vi "SmartSearch.vi"() -> ()   [LabVIEW 2015]
uses:
  <vilib>/NXT/Subs/MotorOutput.ctl
  <vilib>/NXT/Block Support/NXT_InputPort.ctl
  <vilib>/NXT/Dual Mode Library/Sensors/Light_On.vi
  <vilib>/NXT/Dual Mode Library/Motors/MotorReverse.vi
  <vilib>/NXT/Dual Mode Library/Waits/Wait_Num.vi
  <vilib>/NXT/Dual Mode Library/Motors/MotorOn.vi
  <vilib>/NXT/Dual Mode Library/Motors/MotorBrake.vi
  <vilib>/NXT/Dual Mode Library/Sensors/Sonar_cm.vi
panel:
  in  "정지":bool
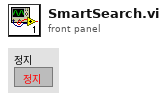
[diagram p1: front panel]
types:
  T1 = typedef "MotorOutput.ctl" = u8
  T2 = typedef "NXT_InputPort.ctl" = u32
  T3 = typedef "LVHSConnector.ctl" = refnum<class "BrickReference.lvclass">
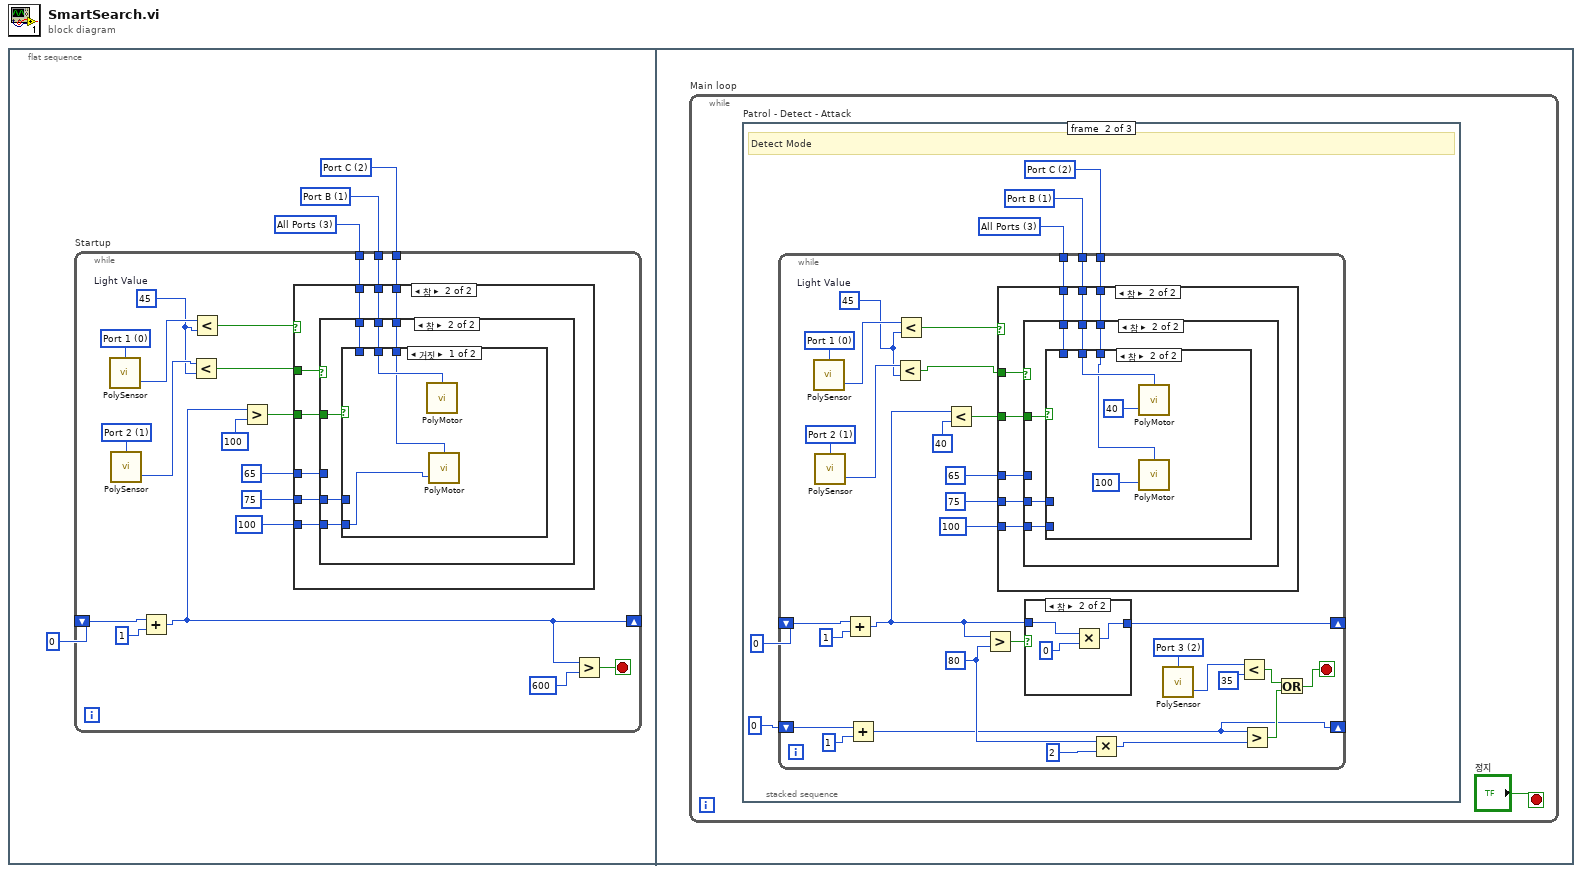
[diagram p0: block diagram]
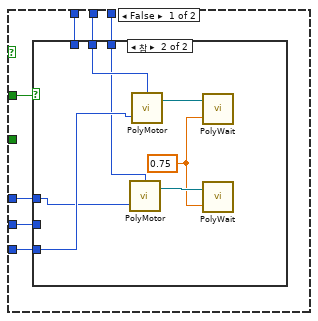
[diagram p2: hidden frame]
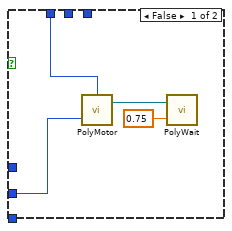
[diagram p3: hidden frame]
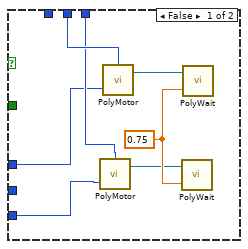
[diagram p4: hidden frame]
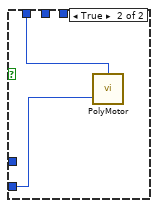
[diagram p5: hidden frame]
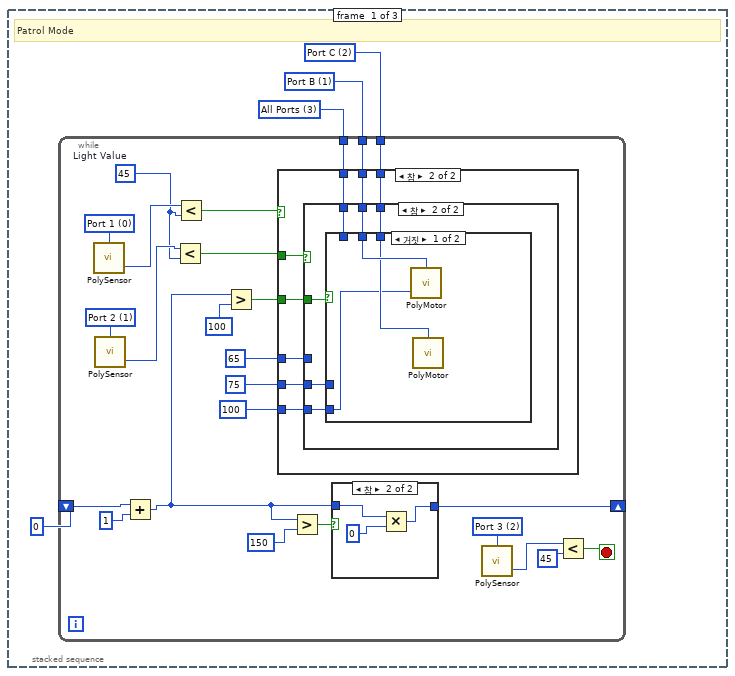
[diagram p6: hidden frame]
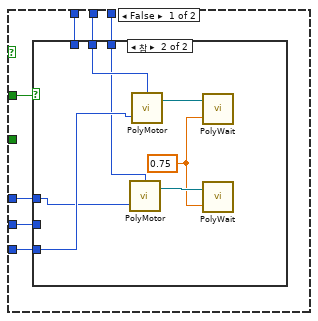
[diagram p8: hidden frame]
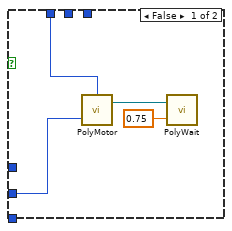
[diagram p9: hidden frame]
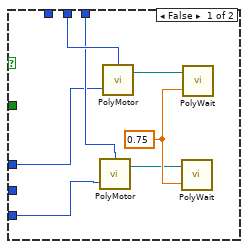
[diagram p10: hidden frame]
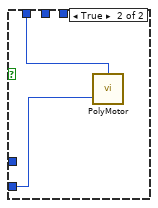
[diagram p11: hidden frame]
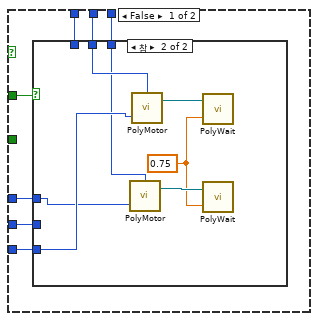
[diagram p13: hidden frame]
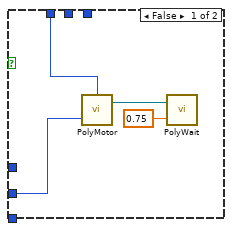
[diagram p14: hidden frame]
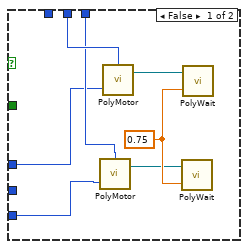
[diagram p15: hidden frame]
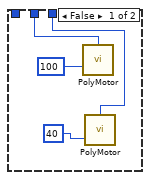
[diagram p16: hidden frame]
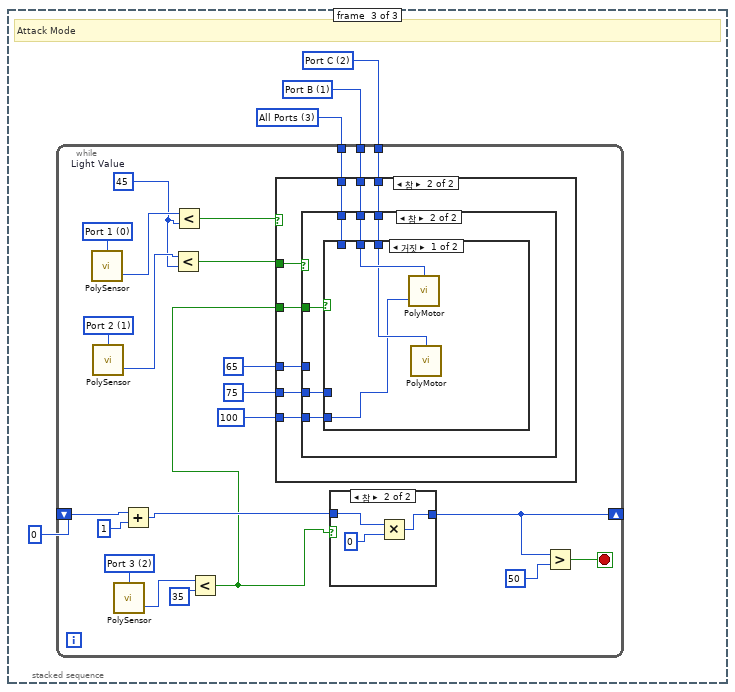
[diagram p17: hidden frame]
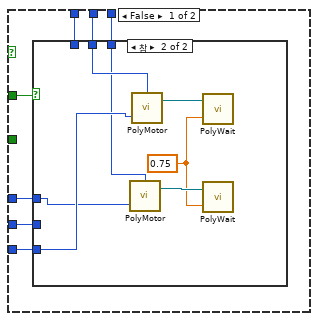
[diagram p19: hidden frame]
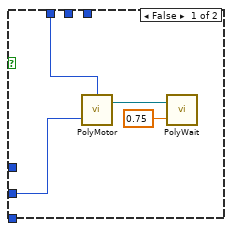
[diagram p20: hidden frame]
diagram:
  n1 = flat-sequence {
    frame #0 {
      w1 = T1 2 items=["Port A"=0, "Port B"=1, "Port C"=2, "Ports A & B"=4, "Ports A & C"=5, "Ports B & C"=6, "All Ports"=3] ("Output Port (All Ports)")
      w2 = T1 1 items=["Port A"=0, "Port B"=1, "Port C"=2, "Ports A & B"=4, "Ports A & C"=5, "Ports B & C"=6, "All Ports"=3] ("Output Port (All Ports)")
      w3 = T1 3 items=["Port A"=0, "Port B"=1, "Port C"=2, "Ports A & B"=4, "Ports A & C"=5, "Ports B & C"=6, "All Ports"=3] ("Output Port (All Ports)")
      n2 = while "Startup" {
        shift-right: [w7] -> _
        shift-left: i16 0 ("y") -> [w12]
        tunnel: w3 -> [w18]
        tunnel: w2 -> [w17]
        tunnel: w1 -> [w16]
        stop <- w6 stop-if-true
        w5 = i16 45  # Light Value
        w22 = T2 1 items=["Port 1", "Port 2", "Port 3", "Port 4"] ("Port (Port 3)")
        w24 = T2 0 items=["Port 1", "Port 2", "Port 3", "Port 4"] ("Port (Port 3)")
        n3 = call-poly <vilib>:"PolySensor.vi"("Port (Port 3)"=w24) -> ("Scaled Value"=w23:i16)  [unwired: 2 in, 1 out]
        n4 = call-poly <vilib>:"PolySensor.vi"("Port (Port 3)"=w22) -> ("Scaled Value"=w21:i16)  [unwired: 2 in, 1 out]
        n5 = Add(x=w12, y=i16 1) -> (x+y=w7:i16)
        n6 = Less?(x=w21, y=w5) -> (x < y?=w8:bool)
        n7 = Less?(x=w23, y=w5) -> (x < y?=w9:bool)
        n8 = Greater?(x=w7, y=i16 100) -> (0:w11:bool)
        n9 = case shown="참" w9 {
          tunnel: w8 -> [w31 w50]
          tunnel: w18 -> [w27 w49]
          tunnel: w17 -> [w26 w48]
          tunnel: w16 -> [w25 w47]
          tunnel: 75 ("Power (75)") -> [w30 w45]
          tunnel: 65 ("Power (75)") -> [w29 w43]
          tunnel: 100 ("Power (75)") -> [w28 w46]
          tunnel: w11 -> [_ w44]
          frame False {
            n10 = case shown="참" w31 {
              tunnel: w30 -> [w34 _]
              tunnel: w29 -> [_ w36]
              tunnel: w28 -> [_ w39]
              tunnel: w27 -> [w32 _]
              tunnel: w26 -> [_ w38]
              tunnel: w25 -> [_ w37]
              frame False {
                n11 = call-poly <vilib>:"PolyMotor.vi"("Power (75)"=w34, "Output Port (All Ports)"=w32) -> ("NXT/EV3"=w33:T3)  [unwired: 1 in, 1 out]
                n12 = call-poly <vilib>:"PolyWait.vi"("Time (1 sec)"=sgl 0.75, "NXT/EV3"=w33) -> ()  [unwired: 2 in, 1 out]
              }
              frame True {
                w40 = sgl 0.75 ("Time (1 sec)")
                n13 = call-poly <vilib>:"PolyMotor.vi"("Power (75)"=w36, "Output Port (All Ports)"=w37) -> ("NXT/EV3"=w41:T3)  [unwired: 1 in, 1 out]
                n14 = call-poly <vilib>:"PolyMotor.vi"("Power (75)"=w39, "Output Port (All Ports)"=w38) -> ("NXT/EV3"=w42:T3)  [unwired: 1 in, 1 out]
                n15 = call-poly <vilib>:"PolyWait.vi"("Time (1 sec)"=w40, "NXT/EV3"=w42) -> ()  [unwired: 2 in, 1 out]
                n16 = call-poly <vilib>:"PolyWait.vi"("Time (1 sec)"=w40, "NXT/EV3"=w41) -> ()  [unwired: 2 in, 1 out]
              }
            }
          }
          frame True {
            n17 = case shown="참" w50 {
              tunnel: w49 -> [_ w63]
              tunnel: w48 -> [w53 w62]
              tunnel: w47 -> [w52 w61]
              tunnel: w46 -> [w54 w59]
              tunnel: w45 -> [_ w60]
              tunnel: w44 -> [_ w58]
              tunnel: w43 -> [w51 _]
              frame False {
                w57 = sgl 0.75 ("Time (1 sec)")
                n18 = call-poly <vilib>:"PolyMotor.vi"("Power (75)"=w54, "Output Port (All Ports)"=w52) -> ("NXT/EV3"=w56:T3)  [unwired: 1 in, 1 out]
                n19 = call-poly <vilib>:"PolyMotor.vi"("Power (75)"=w51, "Output Port (All Ports)"=w53) -> ("NXT/EV3"=w55:T3)  [unwired: 1 in, 1 out]
                n20 = call-poly <vilib>:"PolyWait.vi"("Time (1 sec)"=w57, "NXT/EV3"=w56) -> ()  [unwired: 2 in, 1 out]
                n21 = call-poly <vilib>:"PolyWait.vi"("Time (1 sec)"=w57, "NXT/EV3"=w55) -> ()  [unwired: 2 in, 1 out]
              }
              frame True {
                n22 = case shown="거짓" w58 {
                  tunnel: w63 -> [_ w68]
                  tunnel: w62 -> [w66 _]
                  tunnel: w61 -> [w65 _]
                  tunnel: w60 -> [_ _]
                  tunnel: w59 -> [w64 w67]
                  frame False {
                    n23 = call-poly <vilib>:"PolyMotor.vi"("Port (All Ports)"=w66) -> ()  [unwired: 2 in, 2 out]
                    n24 = call-poly <vilib>:"PolyMotor.vi"("Power (75)"=w64, "Output Port (All Ports)"=w65) -> ()  [unwired: 1 in, 2 out]
                  }
                  frame True {
                    n25 = call-poly <vilib>:"PolyMotor.vi"("Power (75)"=w67, "Output Port (All Ports)"=w68) -> ()  [unwired: 1 in, 2 out]
                  }
                }
              }
            }
          }
        }
        n26 = Greater? ("보다 큼?")(x=w7, y=i16 600) -> (0:w6:bool)
      }
    }
    frame #1 {
      n27 = while "Main loop" {
        stop <- "정지" stop-if-true
        n28 = stacked-sequence "Patrol - Detect - Attack" {
          frame #0 {
            w70 = T1 2 items=["Port A"=0, "Port B"=1, "Port C"=2, "Ports A & B"=4, "Ports A & C"=5, "Ports B & C"=6, "All Ports"=3] ("Output Port (All Ports)")
            w71 = T1 1 items=["Port A"=0, "Port B"=1, "Port C"=2, "Ports A & B"=4, "Ports A & C"=5, "Ports B & C"=6, "All Ports"=3] ("Output Port (All Ports)")
            w72 = T1 3 items=["Port A"=0, "Port B"=1, "Port C"=2, "Ports A & B"=4, "Ports A & C"=5, "Ports B & C"=6, "All Ports"=3] ("Output Port (All Ports)")
            # "Patrol Mode"
            n29 = while {
              shift-right: [w79] -> _
              shift-left: i16 0 ("y") -> [w82]
              tunnel: w72 -> [w88]
              tunnel: w71 -> [w87]
              tunnel: w70 -> [w86]
              stop <- w81 stop-if-true
              w95 = T2 2 items=["Port 1", "Port 2", "Port 3", "Port 4"] ("Port (Port 3)")
              w96 = T2 1 items=["Port 1", "Port 2", "Port 3", "Port 4"] ("Port (Port 3)")
              w93 = i16 45  # Light Value
              w98 = T2 0 items=["Port 1", "Port 2", "Port 3", "Port 4"] ("Port (Port 3)")
              n30 = call-poly <vilib>:"PolySensor.vi"("Port (Port 3)"=w98) -> ("Scaled Value"=w97:i16)  [unwired: 2 in, 1 out]
              n31 = call-poly <vilib>:"PolySensor.vi"("Port (Port 3)"=w96) -> ("Scaled Value"=w94:i16)  [unwired: 2 in, 1 out]
              n32 = Add(x=w82, y=i16 1) -> (x+y=w77:i16)
              n33 = Less?(x=w94, y=w93) -> (x < y?=w74:bool)
              n34 = Less?(x=w97, y=w93) -> (x < y?=w75:bool)
              n35 = Greater?(x=w77, y=i16 100) -> (0:w80:bool)
              n36 = case shown="참" w75 {
                tunnel: w74 -> [w109 w128]
                tunnel: w88 -> [w105 w127]
                tunnel: w87 -> [w104 w126]
                tunnel: w86 -> [w103 w125]
                tunnel: 75 ("Power (75)") -> [w108 w123]
                tunnel: 65 ("Power (75)") -> [w107 w121]
                tunnel: 100 ("Power (75)") -> [w106 w124]
                tunnel: w80 -> [_ w122]
                frame False {
                  n37 = case shown="참" w109 {
                    tunnel: w108 -> [w112 _]
                    tunnel: w107 -> [_ w114]
                    tunnel: w106 -> [_ w117]
                    tunnel: w105 -> [w110 _]
                    tunnel: w104 -> [_ w116]
                    tunnel: w103 -> [_ w115]
                    frame False {
                      n38 = call-poly <vilib>:"PolyMotor.vi"("Power (75)"=w112, "Output Port (All Ports)"=w110) -> ("NXT/EV3"=w111:T3)  [unwired: 1 in, 1 out]
                      n39 = call-poly <vilib>:"PolyWait.vi"("Time (1 sec)"=sgl 0.75, "NXT/EV3"=w111) -> ()  [unwired: 2 in, 1 out]
                    }
                    frame True {
                      w118 = sgl 0.75 ("Time (1 sec)")
                      n40 = call-poly <vilib>:"PolyMotor.vi"("Power (75)"=w114, "Output Port (All Ports)"=w115) -> ("NXT/EV3"=w119:T3)  [unwired: 1 in, 1 out]
                      n41 = call-poly <vilib>:"PolyMotor.vi"("Power (75)"=w117, "Output Port (All Ports)"=w116) -> ("NXT/EV3"=w120:T3)  [unwired: 1 in, 1 out]
                      n42 = call-poly <vilib>:"PolyWait.vi"("Time (1 sec)"=w118, "NXT/EV3"=w120) -> ()  [unwired: 2 in, 1 out]
                      n43 = call-poly <vilib>:"PolyWait.vi"("Time (1 sec)"=w118, "NXT/EV3"=w119) -> ()  [unwired: 2 in, 1 out]
                    }
                  }
                }
                frame True {
                  n44 = case shown="참" w128 {
                    tunnel: w127 -> [_ w141]
                    tunnel: w126 -> [w131 w140]
                    tunnel: w125 -> [w130 w139]
                    tunnel: w124 -> [w132 w137]
                    tunnel: w123 -> [_ w138]
                    tunnel: w122 -> [_ w136]
                    tunnel: w121 -> [w129 _]
                    frame False {
                      w135 = sgl 0.75 ("Time (1 sec)")
                      n45 = call-poly <vilib>:"PolyMotor.vi"("Power (75)"=w132, "Output Port (All Ports)"=w130) -> ("NXT/EV3"=w134:T3)  [unwired: 1 in, 1 out]
                      n46 = call-poly <vilib>:"PolyMotor.vi"("Power (75)"=w129, "Output Port (All Ports)"=w131) -> ("NXT/EV3"=w133:T3)  [unwired: 1 in, 1 out]
                      n47 = call-poly <vilib>:"PolyWait.vi"("Time (1 sec)"=w135, "NXT/EV3"=w134) -> ()  [unwired: 2 in, 1 out]
                      n48 = call-poly <vilib>:"PolyWait.vi"("Time (1 sec)"=w135, "NXT/EV3"=w133) -> ()  [unwired: 2 in, 1 out]
                    }
                    frame True {
                      n49 = case shown="거짓" w136 {
                        tunnel: w141 -> [_ w146]
                        tunnel: w140 -> [w144 _]
                        tunnel: w139 -> [w143 _]
                        tunnel: w138 -> [_ _]
                        tunnel: w137 -> [w142 w145]
                        frame False {
                          n50 = call-poly <vilib>:"PolyMotor.vi"("Power (75)"=w142, "Output Port (All Ports)"=w144) -> ()  [unwired: 1 in, 2 out]
                          n51 = call-poly <vilib>:"PolyMotor.vi"("Port (All Ports)"=w143) -> ()  [unwired: 2 in, 2 out]
                        }
                        frame True {
                          n52 = call-poly <vilib>:"PolyMotor.vi"("Power (75)"=w145, "Output Port (All Ports)"=w146) -> ()  [unwired: 1 in, 2 out]
                        }
                      }
                    }
                  }
                }
              }
              n53 = Greater?(x=w77, y=i16 150) -> (0:w78:bool)
              n54 = case shown="참" w78 {
                tunnel: w77 -> [w99 w102]
                tunnel: [w99 w101] -> w79
                frame False {
                }
                frame True {
                  n55 = Multiply(x=w102, y=i16 0) -> (x*y=w101:i16)
                }
              }
              n56 = call-poly <vilib>:"PolySensor.vi"("Port (Port 4)"=w95) -> ("Distance (cm)"=w92:i16)  [unwired: 2 in, 1 out]
              n57 = Less?(x=w92, y=i16 45) -> (x < y?=w81:bool)
            }
          }
          frame #1 {
            w148 = T1 2 items=["Port A"=0, "Port B"=1, "Port C"=2, "Ports A & B"=4, "Ports A & C"=5, "Ports B & C"=6, "All Ports"=3] ("Output Port (All Ports)")
            w149 = T1 1 items=["Port A"=0, "Port B"=1, "Port C"=2, "Ports A & B"=4, "Ports A & C"=5, "Ports B & C"=6, "All Ports"=3] ("Output Port (All Ports)")
            w150 = T1 3 items=["Port A"=0, "Port B"=1, "Port C"=2, "Ports A & B"=4, "Ports A & C"=5, "Ports B & C"=6, "All Ports"=3] ("Output Port (All Ports)")
            # "Detect Mode"
            n58 = while {
              shift-right: [w166] -> _
              shift-left: i16 0 ("y") -> [w168]
              tunnel: w150 -> [w174]
              tunnel: w149 -> [w173]
              tunnel: w148 -> [w172]
              shift-right: [w156] -> _
              shift-left: i16 0 ("y") -> [w163]
              stop <- w161 stop-if-true
              w152 = i16 45  # Light Value
              w159 = i16 80 ("y")
              w180 = T2 2 items=["Port 1", "Port 2", "Port 3", "Port 4"] ("Port (Port 3)")
              w181 = T2 1 items=["Port 1", "Port 2", "Port 3", "Port 4"] ("Port (Port 3)")
              w183 = T2 0 items=["Port 1", "Port 2", "Port 3", "Port 4"] ("Port (Port 3)")
              n59 = call-poly <vilib>:"PolySensor.vi"("Port (Port 3)"=w183) -> ("Scaled Value"=w182:i16)  [unwired: 2 in, 1 out]
              n60 = call-poly <vilib>:"PolySensor.vi"("Port (Port 3)"=w181) -> ("Scaled Value"=w179:i16)  [unwired: 2 in, 1 out]
              n61 = Add(x=w168, y=i16 1) -> (x+y=w164:i16)
              n62 = Add(x=w163, y=i16 1) -> (x+y=w156:i16)
              n63 = Less?(x=w179, y=w152) -> (x < y?=w153:bool)
              n64 = Less?(x=w182, y=w152) -> (x < y?=w154:bool)
              n65 = Less?(x=w164, y=i16 40) -> (x < y?=w167:bool)
              n66 = Greater?(x=w164, y=w159) -> (0:w165:bool)
              n67 = case shown="참" w154 {
                tunnel: w153 -> [w194 w213]
                tunnel: w174 -> [w190 w212]
                tunnel: w173 -> [w189 w211]
                tunnel: w172 -> [w188 w210]
                tunnel: 75 ("Power (75)") -> [w193 w208]
                tunnel: 65 ("Power (75)") -> [w192 w206]
                tunnel: 100 ("Power (75)") -> [w191 w209]
                tunnel: w167 -> [_ w207]
                frame False {
                  n68 = case shown="참" w194 {
                    tunnel: w193 -> [w197 _]
                    tunnel: w192 -> [_ w199]
                    tunnel: w191 -> [_ w202]
                    tunnel: w190 -> [w195 _]
                    tunnel: w189 -> [_ w201]
                    tunnel: w188 -> [_ w200]
                    frame False {
                      n69 = call-poly <vilib>:"PolyMotor.vi"("Power (75)"=w197, "Output Port (All Ports)"=w195) -> ("NXT/EV3"=w196:T3)  [unwired: 1 in, 1 out]
                      n70 = call-poly <vilib>:"PolyWait.vi"("Time (1 sec)"=sgl 0.75, "NXT/EV3"=w196) -> ()  [unwired: 2 in, 1 out]
                    }
                    frame True {
                      w203 = sgl 0.75 ("Time (1 sec)")
                      n71 = call-poly <vilib>:"PolyMotor.vi"("Power (75)"=w199, "Output Port (All Ports)"=w200) -> ("NXT/EV3"=w204:T3)  [unwired: 1 in, 1 out]
                      n72 = call-poly <vilib>:"PolyMotor.vi"("Power (75)"=w202, "Output Port (All Ports)"=w201) -> ("NXT/EV3"=w205:T3)  [unwired: 1 in, 1 out]
                      n73 = call-poly <vilib>:"PolyWait.vi"("Time (1 sec)"=w203, "NXT/EV3"=w205) -> ()  [unwired: 2 in, 1 out]
                      n74 = call-poly <vilib>:"PolyWait.vi"("Time (1 sec)"=w203, "NXT/EV3"=w204) -> ()  [unwired: 2 in, 1 out]
                    }
                  }
                }
                frame True {
                  n75 = case shown="참" w213 {
                    tunnel: w212 -> [_ w226]
                    tunnel: w211 -> [w216 w225]
                    tunnel: w210 -> [w215 w224]
                    tunnel: w209 -> [w217 w222]
                    tunnel: w208 -> [_ w223]
                    tunnel: w207 -> [_ w221]
                    tunnel: w206 -> [w214 _]
                    frame False {
                      w220 = sgl 0.75 ("Time (1 sec)")
                      n76 = call-poly <vilib>:"PolyMotor.vi"("Power (75)"=w217, "Output Port (All Ports)"=w215) -> ("NXT/EV3"=w219:T3)  [unwired: 1 in, 1 out]
                      n77 = call-poly <vilib>:"PolyMotor.vi"("Power (75)"=w214, "Output Port (All Ports)"=w216) -> ("NXT/EV3"=w218:T3)  [unwired: 1 in, 1 out]
                      n78 = call-poly <vilib>:"PolyWait.vi"("Time (1 sec)"=w220, "NXT/EV3"=w219) -> ()  [unwired: 2 in, 1 out]
                      n79 = call-poly <vilib>:"PolyWait.vi"("Time (1 sec)"=w220, "NXT/EV3"=w218) -> ()  [unwired: 2 in, 1 out]
                    }
                    frame True {
                      n80 = case shown="참" w221 {
                        tunnel: w226 -> [_ _]
                        tunnel: w225 -> [w228 w232]
                        tunnel: w224 -> [w227 w231]
                        tunnel: w223 -> [_ _]
                        tunnel: w222 -> [_ _]
                        frame False {
                          n81 = call-poly <vilib>:"PolyMotor.vi"("Power (75)"=100, "Output Port (All Ports)"=w228) -> ()  [unwired: 1 in, 2 out]
                          n82 = call-poly <vilib>:"PolyMotor.vi"("Power (75)"=40, "Output Port (All Ports)"=w227) -> ()  [unwired: 1 in, 2 out]
                        }
                        frame True {
                          n83 = call-poly <vilib>:"PolyMotor.vi"("Power (75)"=40, "Output Port (All Ports)"=w232) -> ()  [unwired: 1 in, 2 out]
                          n84 = call-poly <vilib>:"PolyMotor.vi"("Power (75)"=100, "Output Port (All Ports)"=w231) -> ()  [unwired: 1 in, 2 out]
                        }
                      }
                    }
                  }
                }
              }
              n85 = case shown="참" w165 {
                tunnel: w164 -> [w184 w187]
                tunnel: [w184 w186] -> w166
                frame False {
                }
                frame True {
                  n86 = Multiply(x=w187, y=i16 0) -> (x*y=w186:i16)
                }
              }
              n87 = Multiply(x=w159, y=i16 2) -> (x*y=w158:i16)
              n88 = call-poly <vilib>:"PolySensor.vi"("Port (Port 4)"=w180) -> ("Distance (cm)"=w178:i16)  [unwired: 2 in, 1 out]
              n89 = Less?(x=w178, y=i16 35) -> (x < y?=w162:bool)
              n90 = Greater? ("보다 큼?")(x=w156, y=w158) -> (0:w157:bool)
              n91 = Or(x=w162, y=w157) -> (x .or. y?=w161:bool)
            }
          }
          frame #2 {
            w238 = T1 2 items=["Port A"=0, "Port B"=1, "Port C"=2, "Ports A & B"=4, "Ports A & C"=5, "Ports B & C"=6, "All Ports"=3] ("Output Port (All Ports)")
            w237 = T1 1 items=["Port A"=0, "Port B"=1, "Port C"=2, "Ports A & B"=4, "Ports A & C"=5, "Ports B & C"=6, "All Ports"=3] ("Output Port (All Ports)")
            w236 = T1 3 items=["Port A"=0, "Port B"=1, "Port C"=2, "Ports A & B"=4, "Ports A & C"=5, "Ports B & C"=6, "All Ports"=3] ("Output Port (All Ports)")
            # "Attack Mode"
            n92 = while {
              shift-right: [w241] -> _
              shift-left: i16 0 ("y") -> [w246]
              tunnel: w236 -> [w252]
              tunnel: w237 -> [w251]
              tunnel: w238 -> [w250]
              stop <- w243 stop-if-true
              w258 = T2 2 items=["Port 1", "Port 2", "Port 3", "Port 4"] ("Port (Port 3)")
              w259 = T2 1 items=["Port 1", "Port 2", "Port 3", "Port 4"] ("Port (Port 3)")
              w256 = i16 45  # Light Value
              w261 = T2 0 items=["Port 1", "Port 2", "Port 3", "Port 4"] ("Port (Port 3)")
              n93 = call-poly <vilib>:"PolySensor.vi"("Port (Port 3)"=w261) -> ("Scaled Value"=w260:i16)  [unwired: 2 in, 1 out]
              n94 = call-poly <vilib>:"PolySensor.vi"("Port (Port 3)"=w259) -> ("Scaled Value"=w257:i16)  [unwired: 2 in, 1 out]
              n95 = call-poly <vilib>:"PolySensor.vi"("Port (Port 4)"=w258) -> ("Distance (cm)"=w255:i16)  [unwired: 2 in, 1 out]
              n96 = Add(x=w246, y=i16 1) -> (x+y=w245:i16)
              n97 = Less?(x=w257, y=w256) -> (x < y?=w239:bool)
              n98 = Less?(x=w260, y=w256) -> (x < y?=w240:bool)
              n99 = Less?(x=w255, y=i16 35) -> (x < y?=w242:bool)
              n100 = case shown="참" w240 {
                tunnel: w239 -> [w272 w291]
                tunnel: w252 -> [w268 w290]
                tunnel: w251 -> [w267 w289]
                tunnel: w250 -> [w266 w288]
                tunnel: 75 ("Power (75)") -> [w271 w286]
                tunnel: 65 ("Power (75)") -> [w270 w284]
                tunnel: 100 ("Power (75)") -> [w269 w287]
                tunnel: w242 -> [_ w285]
                frame False {
                  n101 = case shown="참" w272 {
                    tunnel: w271 -> [w275 _]
                    tunnel: w270 -> [_ w277]
                    tunnel: w269 -> [_ w280]
                    tunnel: w268 -> [w273 _]
                    tunnel: w267 -> [_ w279]
                    tunnel: w266 -> [_ w278]
                    frame False {
                      n102 = call-poly <vilib>:"PolyMotor.vi"("Power (75)"=w275, "Output Port (All Ports)"=w273) -> ("NXT/EV3"=w274:T3)  [unwired: 1 in, 1 out]
                      n103 = call-poly <vilib>:"PolyWait.vi"("Time (1 sec)"=sgl 0.75, "NXT/EV3"=w274) -> ()  [unwired: 2 in, 1 out]
                    }
                    frame True {
                      w281 = sgl 0.75 ("Time (1 sec)")
                      n104 = call-poly <vilib>:"PolyMotor.vi"("Power (75)"=w277, "Output Port (All Ports)"=w278) -> ("NXT/EV3"=w282:T3)  [unwired: 1 in, 1 out]
                      n105 = call-poly <vilib>:"PolyMotor.vi"("Power (75)"=w280, "Output Port (All Ports)"=w279) -> ("NXT/EV3"=w283:T3)  [unwired: 1 in, 1 out]
                      n106 = call-poly <vilib>:"PolyWait.vi"("Time (1 sec)"=w281, "NXT/EV3"=w283) -> ()  [unwired: 2 in, 1 out]
                      n107 = call-poly <vilib>:"PolyWait.vi"("Time (1 sec)"=w281, "NXT/EV3"=w282) -> ()  [unwired: 2 in, 1 out]
                    }
                  }
                }
                frame True {
                  n108 = case shown="참" w291 {
                    tunnel: w290 -> [_ w304]
                    tunnel: w289 -> [w294 w303]
                    tunnel: w288 -> [w293 w302]
                    tunnel: w287 -> [w295 w300]
                    tunnel: w286 -> [_ w301]
                    tunnel: w285 -> [_ w299]
                    tunnel: w284 -> [w292 _]
                    frame False {
                      w298 = sgl 0.75 ("Time (1 sec)")
                      n109 = call-poly <vilib>:"PolyMotor.vi"("Power (75)"=w295, "Output Port (All Ports)"=w293) -> ("NXT/EV3"=w297:T3)  [unwired: 1 in, 1 out]
                      n110 = call-poly <vilib>:"PolyMotor.vi"("Power (75)"=w292, "Output Port (All Ports)"=w294) -> ("NXT/EV3"=w296:T3)  [unwired: 1 in, 1 out]
                      n111 = call-poly <vilib>:"PolyWait.vi"("Time (1 sec)"=w298, "NXT/EV3"=w297) -> ()  [unwired: 2 in, 1 out]
                      n112 = call-poly <vilib>:"PolyWait.vi"("Time (1 sec)"=w298, "NXT/EV3"=w296) -> ()  [unwired: 2 in, 1 out]
                    }
                    frame True {
                      n113 = case shown="거짓" w299 {
                        tunnel: w304 -> [_ w309]
                        tunnel: w303 -> [w307 _]
                        tunnel: w302 -> [w306 _]
                        tunnel: w301 -> [_ _]
                        tunnel: w300 -> [w305 w308]
                        frame False {
                          n114 = call-poly <vilib>:"PolyMotor.vi"("Power (75)"=w305, "Output Port (All Ports)"=w307) -> ()  [unwired: 1 in, 2 out]
                          n115 = call-poly <vilib>:"PolyMotor.vi"("Port (All Ports)"=w306) -> ()  [unwired: 2 in, 2 out]
                        }
                        frame True {
                          n116 = call-poly <vilib>:"PolyMotor.vi"("Power (75)"=w308, "Output Port (All Ports)"=w309) -> ()  [unwired: 1 in, 2 out]
                        }
                      }
                    }
                  }
                }
              }
              n117 = case shown="참" w242 {
                tunnel: w245 -> [w262 w265]
                tunnel: [w262 w264] -> w241
                frame False {
                }
                frame True {
                  n118 = Multiply(x=w265, y=i16 0) -> (x*y=w264:i16)
                }
              }
              n119 = Greater?(x=w241, y=i16 50) -> (0:w243:bool)
            }
          }
        }
      }
    }
  }
